vi "Reset.vi"(8 "error in (no error)":errorcluster, 11 "Counter in":refnum<class "Counter.lvclass">) -> (0 "error out":errorcluster, 3 "Counter out":refnum<class "Counter.lvclass">)   [LabVIEW 2018, in "Counter.lvlib" / "Counter.lvclass"]
uses:
  Counter.lvclass
  Counter.lvclass/Counter.ctl
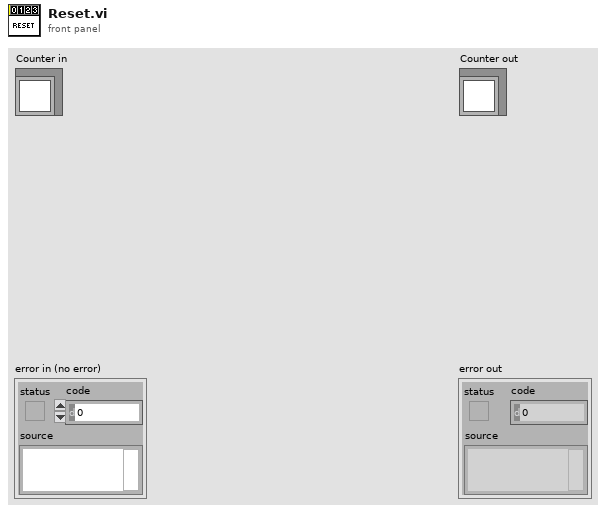
[diagram p1: front panel]
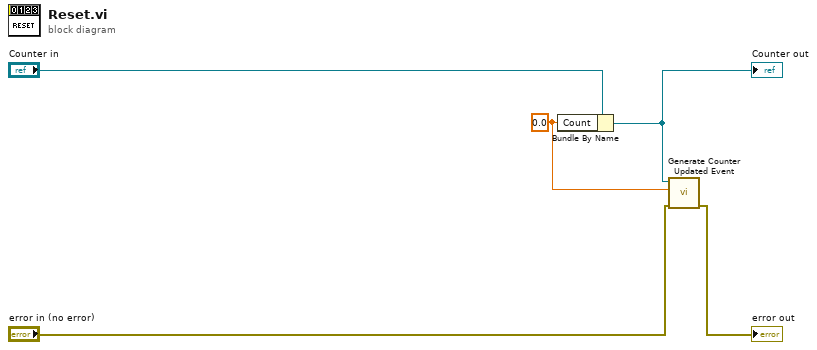
[diagram p0: block diagram]
diagram:
  w3 = 0.0 ("Count")
  n1 = Bundle By Name(cluster="Counter in", "Count"=w3) -> (w4:refnum<class "Counter.lvclass">)
  "Counter out" <- w4
  n2 = call "Generate Counter Updated Event.vi"("error in (no error)"="error in (no error)", "Count"=w3, "Counter in"=w4) -> ("error out"=→"error out":errorcluster)  [unwired: 8 in]
